vi "Attacked.vi"(9 "Team In":refnum<class "Team.lvclass">, 10 "Attackers":T1, 11 "MySquare in":refnum<class "MySquare.lvclass">) -> (1 "Team":refnum<class "Team.lvclass">, 3 "MySquare out":refnum<class "MySquare.lvclass">)   [LabVIEW 2020, in "The_Hill_Youth.lvlib" / "MySquare.lvclass"]
uses:
  MySquare.lvclass
  C:/dev/lv20CE/sol-squarebattle/ProjectTemplates/Source/SummerOfLabVIEW/SquareBattle/template/SquareBattle/Square/Square.lvclass
  SquareBattle/Team/Team.lvclass
  SquareBattle/Attacked Info.ctl
  MyTeam/MyTeam.lvclass
  C:/dev/lv20CE/sol-squarebattle/ProjectTemplates/Source/SummerOfLabVIEW/SquareBattle/template/SquareBattle/Team/Team.lvclass
  MyTeam/map_point.ctl
  SquareBattle/Square/Square.lvclass/Square.ctl
  SquareBattle/Square/Square.lvclass
  SquareBattle/SquareBattle.lvlib
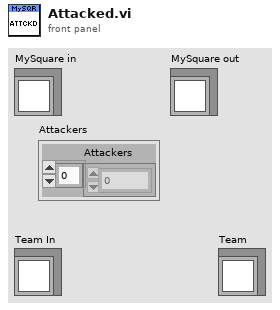
[diagram p1: front panel]
types:
  T1 = typedef "SquareBattle.lvlib/Attacked Info.ctl" = cluster{"Attackers":i32[]}
  T2 = typedef "map_point.ctl" = cluster{"status":enum16{"unknown", "frind", "enemy", "empty"}, "plans":enum16{"stay", "duplicate", "attack", "move to", "no plans"}, "age":dbl}
  T3 = typedef "SquareBattle.lvlib/Position.ctl" = cluster{"Row":i32, "Col":i32}
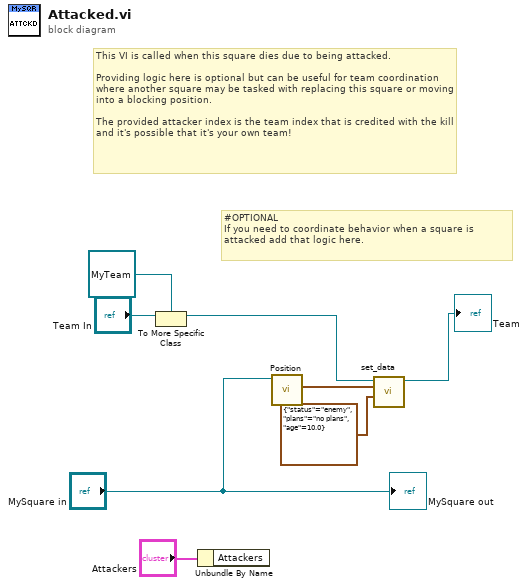
[diagram p0: block diagram]
diagram:
  # "#OPTIONAL\nIf you need to coordinate behavior when a square is attacked add that logic here."
  # "This VI is called when this square dies due to being attacked.\n\nProviding logic here is optional but can be useful for team coordination where another square may be tasked with replacing this square or moving into a blocking position.\n\nThe provided attacker index is the team index that is credited with the kill and it's possible that it's your own team!"
  n1 = To More Specific Class(target class=refnum<class "MyTeam.lvclass"> refnum ("SquareTeam.lvlib:MyTeam.lvclass"), reference="Team In") -> (specific class reference=w3:refnum<class "MyTeam.lvclass">)  [unwired: 1 in, 1 out]
  n2 = Unbundle By Name("Attackers") -> ()  [unwired: 1 out]
  n3 = call "Position.vi"("Square in"="MySquare in") -> ("Position"=w4:T3)  [unwired: 10 in]
  n4 = call "set_data.vi"("new data"=T2 {"status"=enum."enemy", "plans"=enum."no plans", "age"=10.0}, "point to set index"=w4, "SquareTeam.lvlib:MyTeam.lvclass 2"=w3) -> ("SquareTeam.lvlib:MyTeam.lvclass"=→"Team":refnum<class "MyTeam.lvclass">)  [unwired: 8 in]
  "MySquare out" <- "MySquare in"
